vi "Tracing Pass Fail Count.vi"(8 "Result Status":string, 9 "Unique StepId":string, 10 "Test Status":string, 11 "Name":string) -> (0 "Step Result Action":T1(ring), 1 "Fail Count":u32, 2 "Pass Count":u32, 3 "index of element":i32)   [LabVIEW 2023, in "GUI.lvlib"]
uses:
  Global/Global LV.vi
  GUI.lvlib
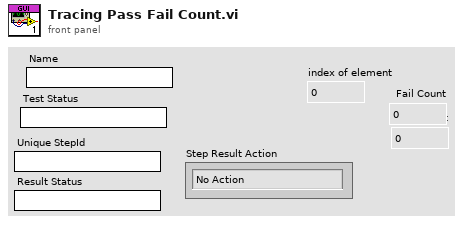
[diagram p1: front panel]
types:
  T1 = enum16{"No Action", "Pass +1", "Fail +1", "Pass +1, Fail -1", "Pass -1, Fail +1"}
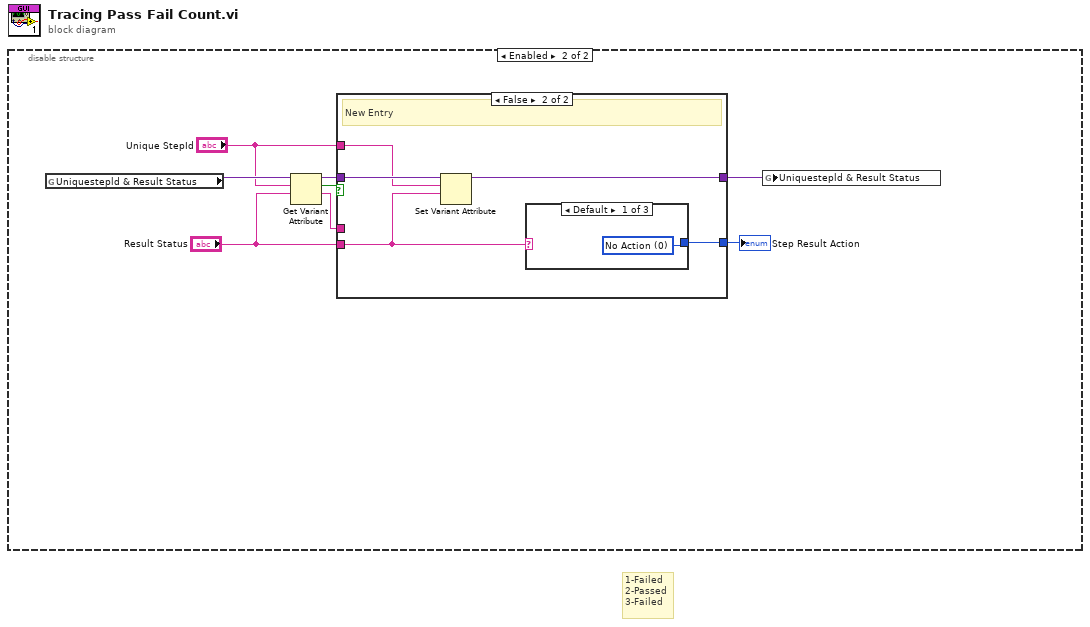
[diagram p0: block diagram]
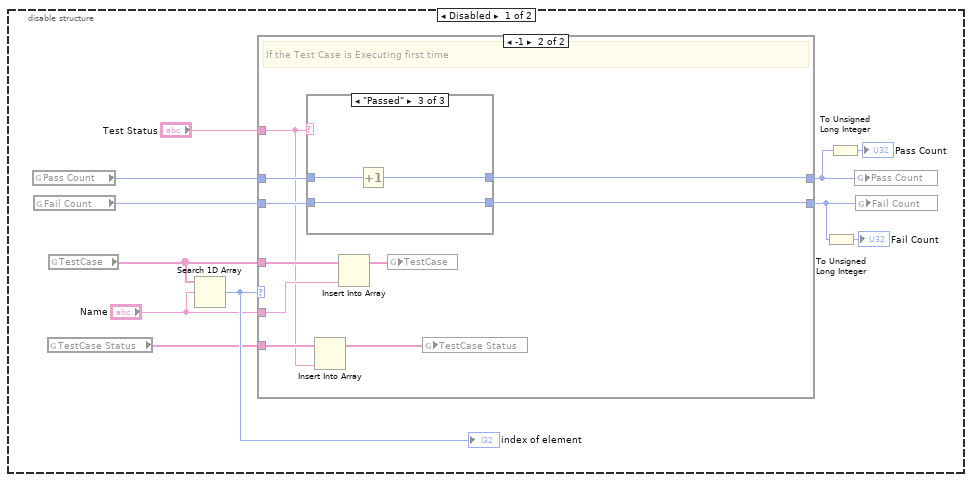
[diagram p2: hidden frame]
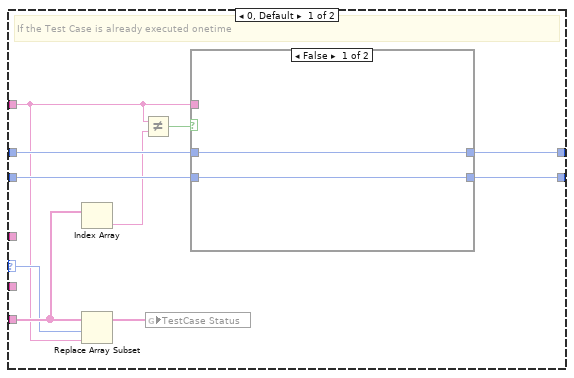
[diagram p3: hidden frame]
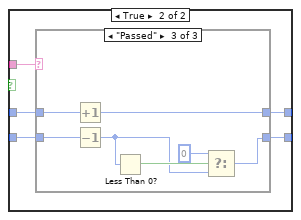
[diagram p4: hidden frame]
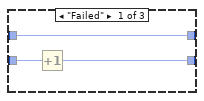
[diagram p7: hidden frame]
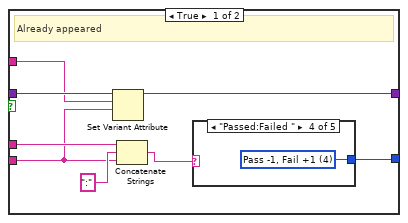
[diagram p9: hidden frame]
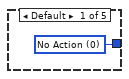
[diagram p10: hidden frame]
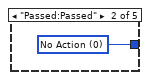
[diagram p11: hidden frame]
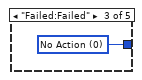
[diagram p12: hidden frame]
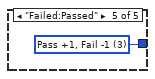
[diagram p13: hidden frame]
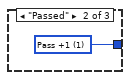
[diagram p14: hidden frame]
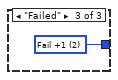
[diagram p15: hidden frame]
diagram:
  # "1-Failed\n2-Passed\n3-Failed"
  n1 = disable-structure shown="Enabled" {
    frame Disabled {
      n2 = global read "Global LV.vi" "Pass Count"() -> (w8:i32)
      n3 = global read "Global LV.vi" "Fail Count"() -> (w7:i32)
      n4 = global read "Global LV.vi" "TestCase Status"() -> (w1:string[])
      n5 = global read "Global LV.vi" "TestCase"() -> (w9:string[])
      n6 = Search 1D Array(1D array=w9, element="Name") -> (index of element=w11:i32)  [unwired: 1 in]
      "index of element" <- w11
      n7 = case shown="-1" w11 {
        selector: w11 -> [w16 _]
        tunnel: "Name" -> [_ w47]
        tunnel: w9 -> [_ w49]
        tunnel: w8 -> [w21 w46]
        tunnel: w7 -> [w20 w45]
        tunnel: "Test Status" -> [w14 w40]
        tunnel: [w19 w44] -> w5
        tunnel: [w18 w43] -> w4
        tunnel: w1 -> [w17 w42]
        frame 0, Default {
          # "If the Test Case is already executed onetime"
          n8 = Index Array(array=w17) -> (element=w13:string)  [unwired: 1 in]
          n9 = Replace Array Subset(array=w17, new element=w14, index=w16) -> (w15:string[])
          n10 = Not Equal?(x=w14, y=w13) -> (x != y?=w12:bool)
          n11 = global write "Global LV.vi" "TestCase Status"(w15) -> ()
          n12 = case shown="False" w12 {
            tunnel: w21 -> [w23 w28]
            tunnel: w20 -> [w22 w27]
            tunnel: [w23 w26] -> w19
            tunnel: [w22 w25] -> w18
            tunnel: w14 -> [_ w24]
            frame False {
            }
            frame True {
              n13 = case shown="\"Passed\"" w24 {
                tunnel: w28 -> [w30 w32 w39]
                tunnel: w27 -> [w29 w31 w37]
                tunnel: [w29 w31 w33] -> w25
                tunnel: [w30 w32 w38] -> w26
                frame "Failed" {
                }
                frame Default {
                }
                frame "Passed" {
                  n14 = Increment(x=w39) -> (x+1=w38:i32)
                  n15 = Decrement(x=w37) -> (x-1=w35:i32)
                  n16 = Less Than 0?(x=w35) -> (x < 0?=w36:bool)
                  n17 = Select(t=0, s=w36, f=w35) -> (s? t:f=w33:i32)
                }
              }
            }
          }
        }
        frame -1 {
          # "If the Test Case is Executing first time"
          n18 = case shown="\"Passed\"" w40 {
            tunnel: w46 -> [w50 w54 w57]
            tunnel: w45 -> [w52 w53 w55]
            tunnel: [w51 w53 w55] -> w43
            tunnel: [w50 w54 w56] -> w44
            frame "Failed" {
              n19 = Increment(x=w52) -> (x+1=w51:i32)
            }
            frame Default {
            }
            frame "Passed" {
              n20 = Increment(x=w57) -> (x+1=w56:i32)
            }
          }
          n21 = Insert Into Array(array=w42, new element=w40) -> (w41:string[])  [unwired: 1 in]
          n22 = Insert Into Array(array=w49, new element=w47) -> (w48:string[])  [unwired: 1 in]
          n23 = global write "Global LV.vi" "TestCase"(w48) -> ()
          n24 = global write "Global LV.vi" "TestCase Status"(w41) -> ()
        }
      }
      n25 = To Unsigned Long Integer(number=w4) -> (unsigned 32bit integer=→"Fail Count":u32)
      n26 = To Unsigned Long Integer(number=w5) -> (unsigned 32bit integer=→"Pass Count":u32)
      n27 = global write "Global LV.vi" "Pass Count"(w5) -> ()
      n28 = global write "Global LV.vi" "Fail Count"(w4) -> ()
    }
    frame Enabled {
      n29 = global read "Global LV.vi" "Uniquestepld & Result Status"() -> (w65:variant)
      n30 = Get Variant Attribute(Variant=w65, name="Unique StepId", default value (empty Variant)="Result Status") -> (duplicate Variant=w64:variant, found=w63:bool, value=w62:string)  [unwired: 1 in, 1 out]
      n31 = case shown="False" w63 {
        tunnel: w64 -> [w73 w83]
        tunnel: w62 -> [w72 _]
        tunnel: "Result Status" -> [w69 w80]
        tunnel: "Unique StepId" -> [w70 w82]
        tunnel: [w68 w81] -> w59
        tunnel: [w66 w79] -> w58
        frame True {
          # "Already appeared"
          n32 = Set Variant Attribute(Variant=w73, name=w70, value=w69) -> (Variant out=w68:variant)  [unwired: 1 in, 2 out]
          n33 = Concatenate Strings(w72, ":" ("string"), w69) -> (w67:string)
          n34 = case shown="\"Passed:Failed \"" w67 {
            tunnel: [w74 w75 w76 w77 w78] -> w66
            frame Default {
              w74 = u16 0 items=["No Action", "Pass +1", "Fail +1", "Pass +1, Fail -1", "Pass -1, Fail +1"] ("Step Result Action")
            }
            frame "Passed:Passed" {
              w75 = u16 0 items=["No Action", "Pass +1", "Fail +1", "Pass +1, Fail -1", "Pass -1, Fail +1"] ("Step Result Action")
            }
            frame "Failed:Failed" {
              w76 = u16 0 items=["No Action", "Pass +1", "Fail +1", "Pass +1, Fail -1", "Pass -1, Fail +1"] ("Step Result Action")
            }
            frame "Passed:Failed " {
              w77 = u16 4 items=["No Action", "Pass +1", "Fail +1", "Pass +1, Fail -1", "Pass -1, Fail +1"] ("Step Result Action")
            }
            frame "Failed:Passed" {
              w78 = u16 3 items=["No Action", "Pass +1", "Fail +1", "Pass +1, Fail -1", "Pass -1, Fail +1"] ("Step Result Action")
            }
          }
        }
        frame False {
          # "New Entry"
          n35 = Set Variant Attribute(Variant=w83, name=w82, value=w80) -> (Variant out=w81:variant)  [unwired: 1 in, 2 out]
          n36 = case shown="Default" w80 {
            tunnel: [w84 w85 w86] -> w79
            frame Default {
              w84 = u16 0 items=["No Action", "Pass +1", "Fail +1", "Pass +1, Fail -1", "Pass -1, Fail +1"] ("Step Result Action")
            }
            frame "Passed" {
              w85 = u16 1 items=["No Action", "Pass +1", "Fail +1", "Pass +1, Fail -1", "Pass -1, Fail +1"] ("Step Result Action")
            }
            frame "Failed" {
              w86 = u16 2 items=["No Action", "Pass +1", "Fail +1", "Pass +1, Fail -1", "Pass -1, Fail +1"] ("Step Result Action")
            }
          }
        }
      }
      "Step Result Action" <- w58
      n37 = global write "Global LV.vi" "Uniquestepld & Result Status"(w59) -> ()
    }
  }
